vi "Configure Lamp State.vi"(8 "error in (no error)":errorcluster, 10 "state":u16(ring)=1 items=["off"=0, "on"=1, "pulses"=3], 11 "Lotis in":refnum<class "PL Lotis TII LS.lvclass">) -> (0 "error out":errorcluster, 3 "Lotis out":refnum<class "PL Lotis TII LS.lvclass">)   [LabVIEW 2015, in "PL Lotis TII LS.lvclass"]
doc: "Configures lamp state."
uses:
  PL Lotis TII LS.lvclass
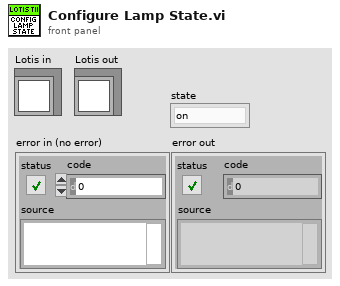
[diagram p1: front panel]
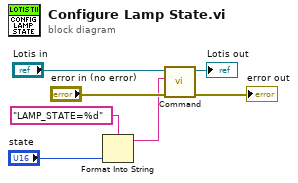
[diagram p0: block diagram]
diagram:
  n1 = Format Into String(format string="LAMP_STATE=%d" ("command"), "state") -> (resulting string=w2:string)  [unwired: 2 in, 1 out]
  n2 = call "Command.vi"("error in (no error)"="error in (no error)", "command"=w2, "Lotis in"="Lotis in") -> ("error out"=→"error out":errorcluster, "Lotis out"=→"Lotis out":refnum<class "PL Lotis TII LS.lvclass">)  [unwired: 6 in, 1 out]
